vi "Length_5_R2.vi"() -> ()   [LabVIEW 2020]
uses:
  Support/Controls/Clst_Initialize Input.ctl
  Support/Controls/Clst_Result inspec.ctl
  Support/Controls/Cmd_Var Data IO.ctl
  Support/Controls/Cmd_Mouse Popup.ctl
  Variables/Global_Cal Info.vi
panel:
  in  "Measured 2":string[][](table) caption="잔류잡음측정"
  in  "Measured_ADJ":string[][](table) caption="조정후"
  out "최소범위":string
  in  "표시방식":string(combo)
  out "단위":string
  out "최대범위":string
  in  "Spec 변경":bool
  in  "Random":bool
  out "Resolution":string[][](table) caption="Spec"
  out "Spec":string[][](table)
  out "제목":string
  out "에러 출력":errorcluster
  out "Condition":string[][](table) caption="2. 직선성 시험"
  in  "최소눈금":string(combo)
  in  "Measured":string[][](table) caption="조정전"
  out "Load?":bool
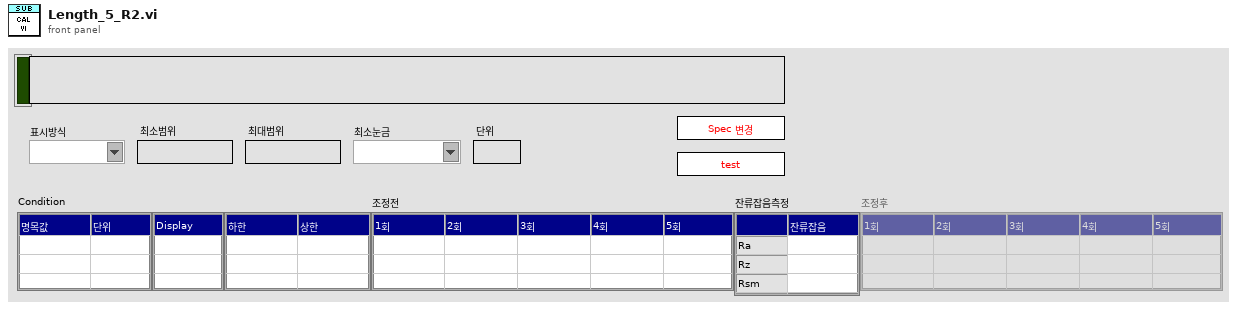
[diagram p1: front panel]
types:
  T1 = typedef "Cmd_Mouse Popup.ctl" = enum16{"활성화", "메뉴선택"}
  T2 = cluster{"Shift":bool, "Ctrl":bool, "Alt":bool, "Cmd":bool, "Opt":bool}
  T3 = typedef "Clst_Initialize Input.ctl" = cluster{"Initialize 1":cluster{"Condition":refnum<vi>[], "Spec":refnum<vi>[], "Measured":refnum<vi>[], "Resolution":refnum<vi>[], "Func_ext":string, "제목":refnum<vi>, "Measured_ADJ":refnum<vi>[]}, "Initialize 2":cluster{"문자열":refnum<vi>[], "콤보박스":refnum<vi>[], "링":refnum<vi>[], "열거형":refnum<vi>[], "테이블":refnum<vi>[], "여러열":refnum<vi>[], "디지털(DBL)":refnum<vi>[], "3D string":refnum<vi>[], "ctrl":refnum<vi>[], "boolean":refnum<vi>[]}}
  T4 = typedef "Clst_Result inspec.ctl" = cluster{"분해능":string, "문자열 1":string, "문자열 2":string, "숫자형 1":i32, "숫자형 2":i32, "숫자형 3":dbl, "문자배열 1D":string[], "문자배열 2D":string[][], "문자배열 3D":string[][][], "문자배열 4D":string[][][][], "불리언 1D":bool[]}
  T5 = typedef "Cmd_Var Data IO.ctl" = enum16{"Condition", "Condition Default", "Condition_Temp", "Resolution", "Resolution Default", "Resolution Old", "Spec", "Spec Default", "Spec Old", "Spec Temp", "Result", "Result2", "Result3", "Result_Temp", "Result_ADJ", "Result_ADJ2", "STD1", "STD2", "STD3", "STD4", "STD5", "STD Temp", "CMC", "CMC Default"}
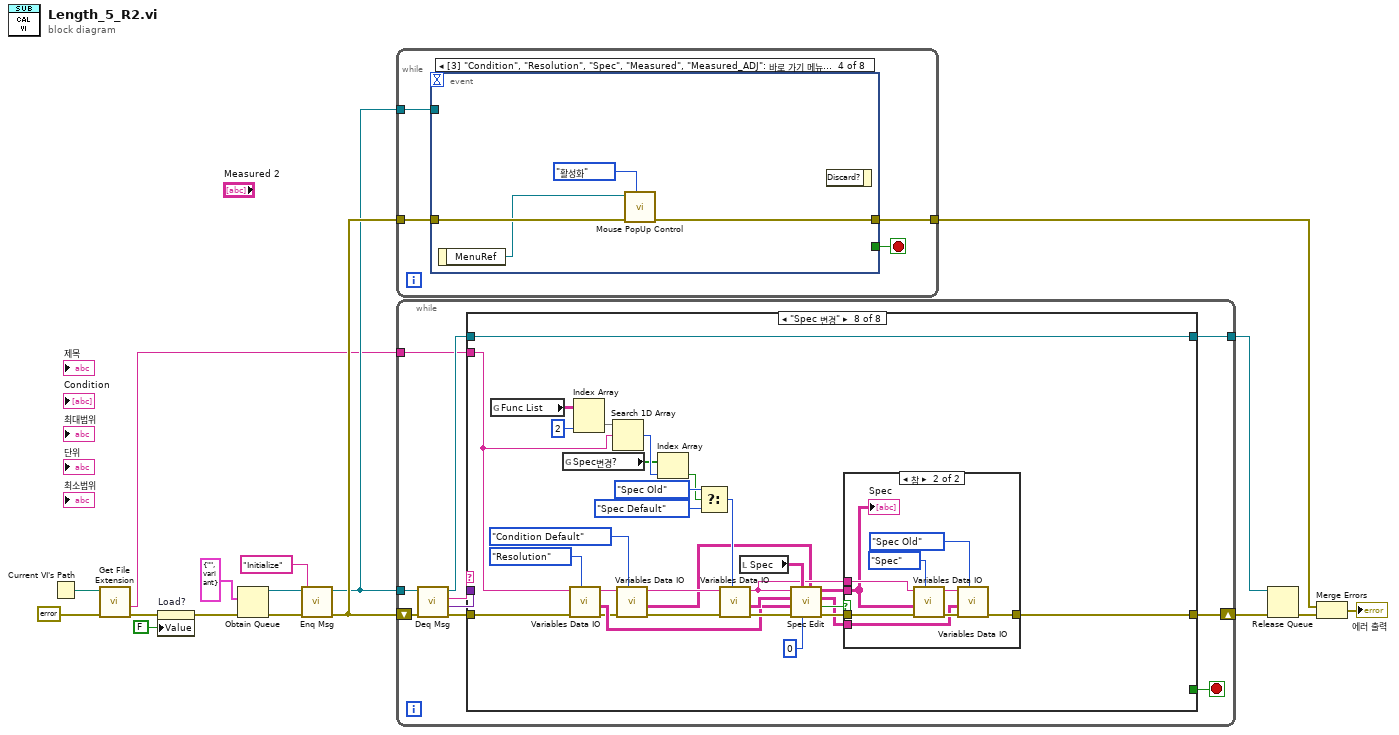
[diagram p0: block diagram]
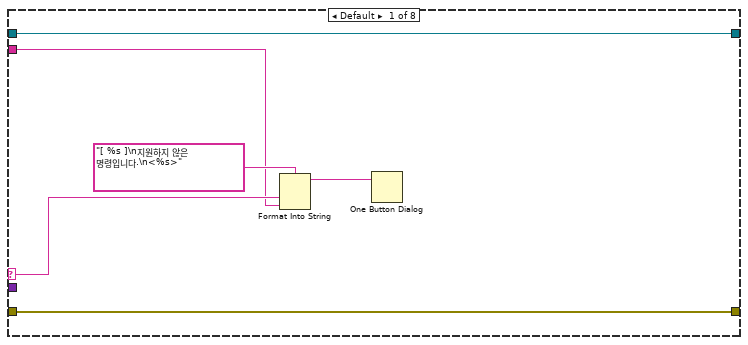
[diagram p2: hidden frame]
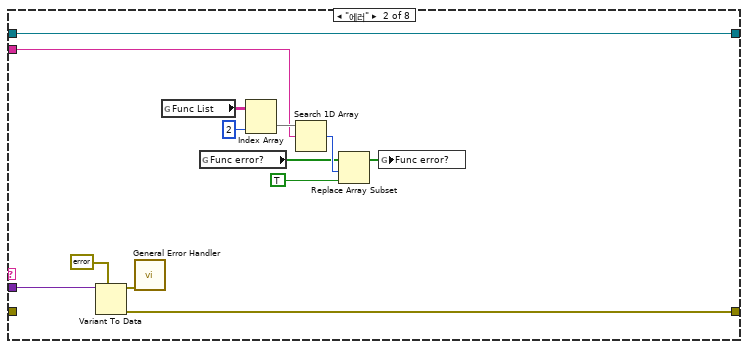
[diagram p3: hidden frame]
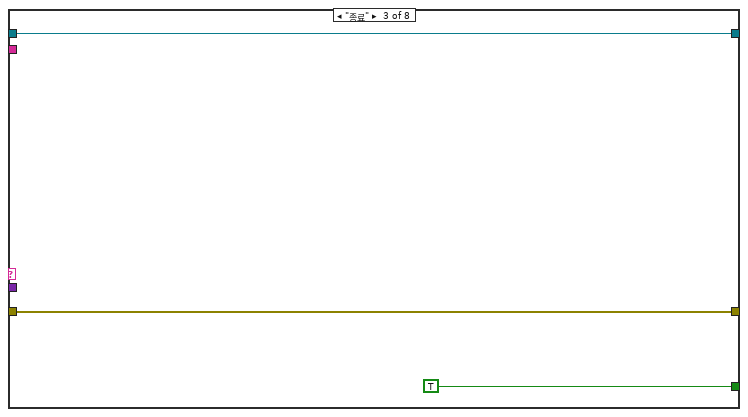
[diagram p4: hidden frame]
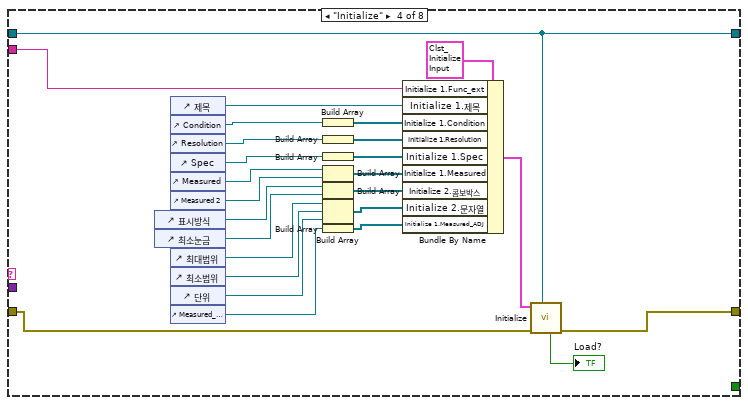
[diagram p5: hidden frame]
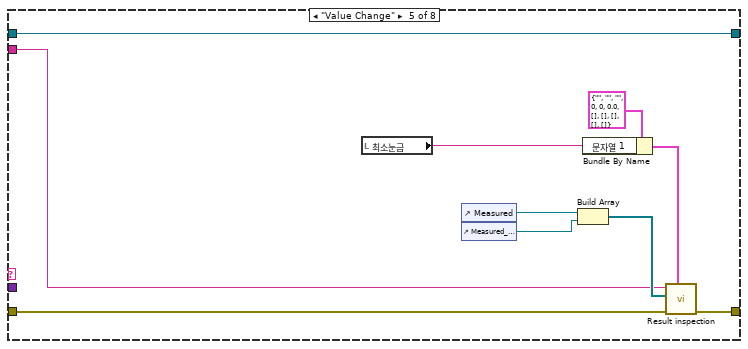
[diagram p6: hidden frame]
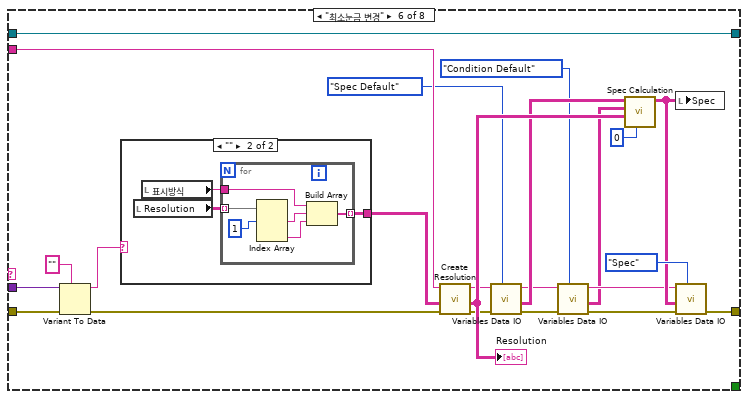
[diagram p7: hidden frame]
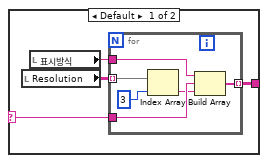
[diagram p8: hidden frame]
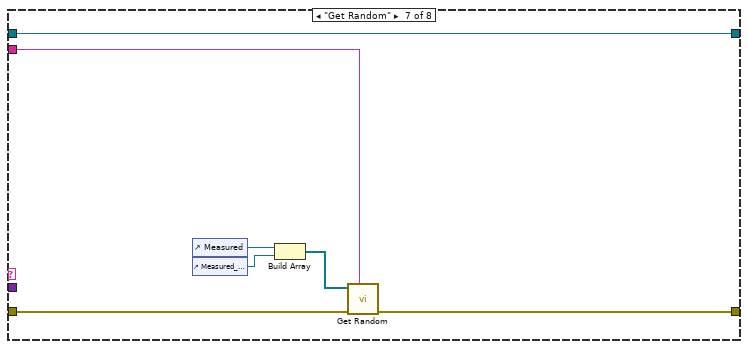
[diagram p9: hidden frame]
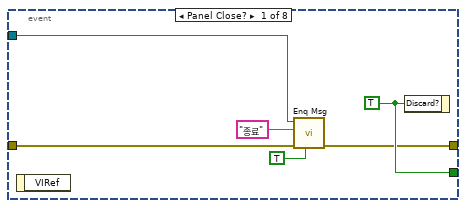
[diagram p11: hidden frame]
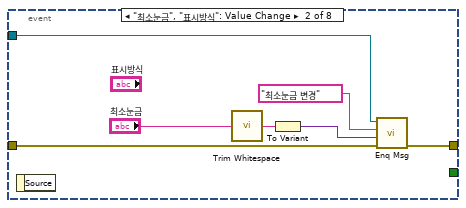
[diagram p12: hidden frame]
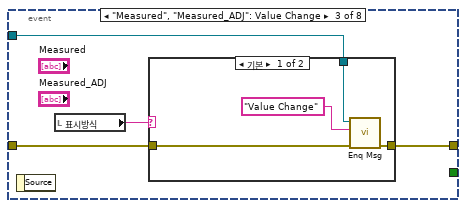
[diagram p13: hidden frame]
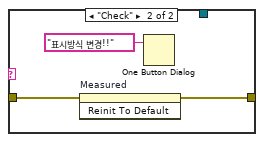
[diagram p14: hidden frame]
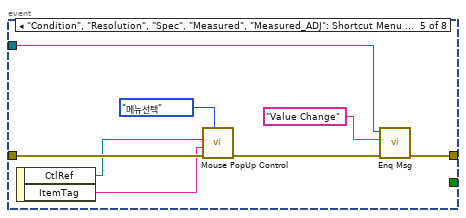
[diagram p15: hidden frame]
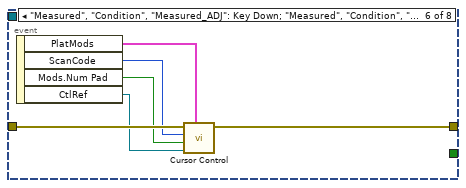
[diagram p16: hidden frame]
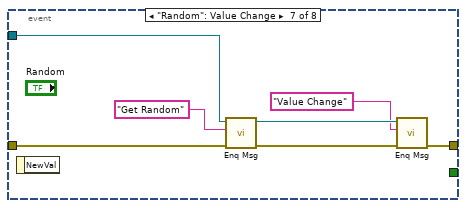
[diagram p17: hidden frame]
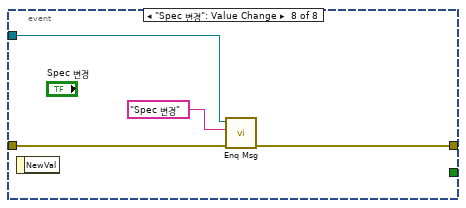
[diagram p18: hidden frame]
diagram:
  n1 = Current VI's Path() -> (path=w5:path)
  n2 = call <vilib>:"Get File Extension.vi"("error in (no error)"=errorcluster {"status"=FALSE, "code"=0, "source"=""} ("에러 상수"), "file"=w5) -> ("error out"=w3:errorcluster, "filename without extension"=w4:string)  [unwired: 5 in, 3 out]
  n3 = property on="Load?" class="Bool (엄격한)"(error in=w3, "Value"=FALSE ("Load?")) -> (error out=w2:errorcluster)  [unwired: 1 in, 1 out]
  n4 = Obtain Queue(element data type=cluster{"메세지":string, "값":variant} {"메세지"="", "값"=variant} ("Message Cluster"), error in (no error)=w2) -> (queue out=w14:refnum<queue>, error out=w16:errorcluster)  [unwired: 3 in, 1 out]
  n5 = call "Enq Msg.vi"("에러 입력(에러 없음)"=w16, "메세지"="Initialize", "큐 입력"=w14) -> ("에러 출력"=w15:errorcluster, "큐 출력"=w12:refnum<queue>)  [unwired: 7 in]
  n6 = while {
    tunnel: w15 -> [w19]
    tunnel: w12 -> [w20]
    tunnel: [w18] -> w9
    stop <- w21 stop-if-true
    n7 = event shown="[3] \"Condition\", \"Resolution\", \"Spec\", \"Measured\", \"Measured_ADJ\": 바로 가기 메뉴 활성화?" {
      selector: _ -> [_ _ _ _ _ _ _ _]
      dyn-events: _ -> [_ _ _ _ _ _ _ _]
      timeout: _ -> [_ _ _ _ _ _ _ _]
      tunnel: [w27 _ _ _ _ _ _ _] -> w21
      tunnel: w20 -> [w25 w33 w38 _ w50 _ w68 w72]
      tunnel: w19 -> [w26 w34 w36 w49 w57 w63 w69 w73]
      tunnel: [w23 w32 w37 w48 w51 w62 w64 w71] -> w18
      event Panel Close? {
        w27 = TRUE ("버림?")
        n8 = event-data() -> ()  [unwired: 1 in, 1 out]
        n9 = call "Enq Msg.vi"("우선순위 메시지?"=TRUE, "에러 입력(에러 없음)"=w26, "메세지"="종료", "큐 입력"=w25) -> ("에러 출력"=w23:errorcluster)  [unwired: 6 in, 1 out]
        n10 = event-data("Discard?"=w27) -> ()  [unwired: 1 in, 1 out]
      }
      event "최소눈금", "표시방식": Value Change {
        n11 = event-data() -> ()  [unwired: 1 in, 1 out]
        n12 = call <vilib>:"Trim Whitespace.vi"("string"="최소눈금") -> ("trimmed string"=w30:string)  [unwired: 1 in]
        n13 = To Variant(anything=w30) -> (Variant=w28:variant)
        n14 = call "Enq Msg.vi"("에러 입력(에러 없음)"=w34, "값"=w28, "메세지"="최소눈금 변경", "큐 입력"=w33) -> ("에러 출력"=w32:errorcluster)  [unwired: 6 in, 1 out]
      }
      event "Measured", "Measured_ADJ": Value Change {
        n15 = event-data() -> ()  [unwired: 1 in, 1 out]
        n16 = local read "표시방식"() -> (w35:string)
        n17 = case shown="기본" w35 {
          tunnel: w38 -> [w42 _]
          tunnel: [w41 w43] -> w37
          tunnel: w36 -> [w40 w44]
          frame Default {
            n18 = call "Enq Msg.vi"("에러 입력(에러 없음)"=w40, "메세지"="Value Change", "큐 입력"=w42) -> ("에러 출력"=w41:errorcluster)  [unwired: 7 in, 1 out]
          }
          frame "Check" {
            n19 = invoke on="Measured" class="Tbl (엄격한)" method="Reinit To Default"(error in=w44) -> (error out=w43:errorcluster)  [unwired: 2 in, 2 out]
            n20 = One Button Dialog(message="표시방식 변경!!" ("메시지")) -> ()  [unwired: 1 in, 1 out]
          }
        }
      }
      event "Condition", "Resolution", "Spec", "Measured", "Measured_ADJ": Shortcut Menu Activation? {
        n21 = event-data() -> ("MenuRef"=w47:refnum<k9>)  [unwired: 1 in]
        n22 = call "Mouse PopUp Control.vi"("type"=Cmd_Mouse_Popup."활성화", "error in"=w49, "메뉴 참조"=w47) -> ("error out"=w48:errorcluster)  [unwired: 8 in]
        n23 = event-data() -> ()  [unwired: 2 in, 1 out]
      }
      event "Condition", "Resolution", "Spec", "Measured", "Measured_ADJ": Shortcut Menu Selection (User) {
        n24 = event-data() -> ("CtlRef"=w55:refnum<vi>, "ItemTag"=w54:string)  [unwired: 1 in]
        n25 = call "Mouse PopUp Control.vi"("type"=Cmd_Mouse_Popup."메뉴선택", "error in"=w57, "아이템 태그"=w54, "Tbl 참조 번호"=w55) -> ("error out"=w52:errorcluster)  [unwired: 7 in]
        n26 = call "Enq Msg.vi"("에러 입력(에러 없음)"=w52, "메세지"="Value Change", "큐 입력"=w50) -> ("에러 출력"=w51:errorcluster)  [unwired: 7 in, 1 out]
      }
      event "Measured", "Condition", "Measured_ADJ": Key Down; "Measured", "Condition", "Measured_ADJ": Key Repeat {
        n27 = event-data() -> ("PlatMods"=w58:T2, "ScanCode"=w61:i16, "Mods.Num Pad"=w60:bool, "CtlRef"=w59:refnum<vi>)  [unwired: 1 in]
        n28 = call "Cursor Control.vi"("플랫폼 조합키"=w58, "참조"=w59, "Num Pad"=w60, "ScanCode"=w61, "error in"=w63) -> ("error out"=w62:errorcluster)  [unwired: 5 in, 1 out]
      }
      event "Random": Value Change {
        n29 = event-data() -> ()  [unwired: 1 in, 1 out]
        n30 = call "Enq Msg.vi"("에러 입력(에러 없음)"=w69, "메세지"="Get Random", "큐 입력"=w68) -> ("에러 출력"=w67:errorcluster, "큐 출력"=w66:refnum<queue>)  [unwired: 7 in]
        n31 = call "Enq Msg.vi"("에러 입력(에러 없음)"=w67, "메세지"="Value Change", "큐 입력"=w66) -> ("에러 출력"=w64:errorcluster)  [unwired: 7 in, 1 out]
      }
      event "Spec 변경": Value Change {
        n32 = event-data() -> ()  [unwired: 1 in, 1 out]
        n33 = call "Enq Msg.vi"("에러 입력(에러 없음)"=w73, "메세지"="Spec 변경", "큐 입력"=w72) -> ("에러 출력"=w71:errorcluster)  [unwired: 7 in, 1 out]
      }
    }
  }
  n34 = while {
    shift-right: [w84] -> w11
    shift-left: w15 -> [w83]
    tunnel: w12 -> [w81]
    tunnel: [w76] -> w10
    tunnel: w4 -> [w75]
    stop <- w77 stop-if-true
    n35 = call "Deq Msg.vi"("에러 입력(에러 없음)"=w83, "큐 입력"=w81) -> ("에러 출력"=w82:errorcluster, "값"=w78:variant, "메세지"=w80:string, "큐 출력"=w79:refnum<queue>)  [unwired: 6 in]
    n36 = case shown="\"Spec 변경\"" w80 {
      selector: w80 -> [w86 _ _ _ _ _ _ _]
      tunnel: w82 -> [w90 _ w106 w132 w136 w164 w187 w214]
      tunnel: [w90 w100 w106 w122 w141 w157 w188 w217] -> w84
      tunnel: w79 -> [w89 w99 w104 w116 w142 w165 w191 w221]
      tunnel: w78 -> [_ w101 _ _ _ w163 _ _]
      tunnel: [_ _ TRUE ("버림?") _ _ _ _ _] -> w77
      tunnel: [w89 w99 w104 w116 w142 w165 w191 w221] -> w76
      tunnel: w75 -> [w85 w91 _ w117 w135 w161 w186 w199]
      frame Default {
        n37 = Format Into String(format string="[ %s ]\n지원하지 않은 명령입니다.\n<%s>" ("메시지"), w86, w85) -> (resulting string=w87:string)  [unwired: 2 in, 1 out]
        n38 = One Button Dialog(message=w87) -> ()  [unwired: 1 in, 1 out]
      }
      frame "에러" {
        n39 = Variant To Data(type=errorcluster {"status"=FALSE, "code"=0, "source"=""} ("에러 출력"), Variant=w101) -> (data=w103:errorcluster, error out=w100:errorcluster)  [unwired: 1 in]
        n40 = call <vilib>:"General Error Handler.vi"("error in (no error)"=w103) -> ()  [unwired: 10 in, 5 out]
        n41 = global read "Global_Cal Info.vi" "Func List"() -> (w93:string[][])
        n42 = global read "Global_Cal Info.vi" "Func error?"() -> (w96:bool[])
        n43 = Index Array(array=w93, index (col)=2 ("비활성화된 인덱스 (열)")) -> (element=w94:string[])  [unwired: 1 in]
        n44 = Search 1D Array(1D array=w94, element=w91) -> (index of element=w97:i32)  [unwired: 1 in]
        n45 = Replace Array Subset(array=w96, new element=TRUE ("새 원소/부분배열"), index=w97) -> (w98:bool[])
        n46 = global write "Global_Cal Info.vi" "Func error?"(w98) -> ()
      }
      frame "종료" {
      }
      frame "Initialize" {
        n47 = control-ref of="표시방식"() -> (w115:refnum<vi>)
        n48 = control-ref of="최소눈금"() -> (w125:refnum<vi>)
        n49 = control-ref of="제목"() -> (w123:refnum<vi>)
        n50 = control-ref of="Condition"() -> (w129:refnum<vi>)
        n51 = control-ref of="Resolution"() -> (w118:refnum<vi>)
        n52 = control-ref of="Spec"() -> (w121:refnum<vi>)
        n53 = control-ref of="Measured"() -> (w126:refnum<vi>)
        n54 = control-ref of="Measured 2"() -> (w107:refnum<vi>)
        n55 = control-ref of="최대범위"() -> (w111:refnum<vi>)
        n56 = control-ref of="최소범위"() -> (w112:refnum<vi>)
        n57 = control-ref of="단위"() -> (w114:refnum<vi>)
        n58 = control-ref of="Measured_ADJ"() -> (w109:refnum<vi>)
        n59 = Build Array(w129) -> (w128:refnum<vi>[])
        n60 = Build Array(w118) -> (w119:refnum<vi>[])
        n61 = Build Array(w121) -> (w120:refnum<vi>[])
        n62 = Build Array(w126, w107) -> (w127:refnum<vi>[])
        n63 = Build Array(w115, w125) -> (w124:refnum<vi>[])
        n64 = Build Array(w111, w112, w114) -> (w113:refnum<vi>[])
        n65 = Build Array(w109) -> (w108:refnum<vi>[])
        n66 = Bundle By Name(cluster=T3 {"Initialize 1"={"Condition"=[], "Spec"=[], "Measured"=[], "Resolution"=[], "Func_ext"="", "제목"=refnum, "Measured_ADJ"=[]}, "Initialize 2"={"문자열"=[], "콤보박스"=[], "링"=[], "열거형"=[], "테이블"=[], "여러열"=[], "디지털(DBL)"=[], "3D string"=[], "ctrl"=[], "boolean"=[]}} ("입력 클러스터"), "Initialize 1.Func_ext"=w117, "Initialize 1.제목"=w123, "Initialize 1.Condition"=w128, "Initialize 1.Resolution"=w119, "Initialize 1.Spec"=w120, "Initialize 1.Measured"=w127, "Initialize 2.콤보박스"=w124, "Initialize 2.문자열"=w113, "Initialize 1.Measured_ADJ"=w108) -> (w130:T3)
        n67 = call "Initialize.vi"("큐 입력"=w116, "error in"=w132, "입력 클러스터"=w130) -> ("error out"=w122:errorcluster, "Load?"=→"Load?":bool)  [unwired: 5 in, 2 out]
      }
      frame "Value Change" {
        n68 = local read "최소눈금"() -> (w134:string)
        n69 = control-ref of="Measured"() -> (w140:refnum<vi>)
        n70 = control-ref of="Measured_ADJ"() -> (w133:refnum<vi>)
        n71 = Build Array(w140, w133) -> (w139:refnum<vi>[])
        n72 = Bundle By Name(cluster=T4 {"분해능"="", "문자열 1"="", "문자열 2"="", "숫자형 1"=0, "숫자형 2"=0, "숫자형 3"=0.0, "문자배열 1D"=[], "문자배열 2D"=[], "문자배열 3D"=[], "문자배열 4D"=[], "불리언 1D"=[]} ("입력 클러스터"), "문자열 1"=w134) -> (w137:T4)
        n73 = call "Result inspection.vi"("입력 클러스터"=w137, "error in"=w136, "Ref. Data (Inspection)"=w139, "Func ext"=w135) -> ("error out"=w141:errorcluster)  [unwired: 4 in, 3 out]
      }
      frame "최소눈금 변경" {
        n74 = Variant To Data(error in=w164, type="", Variant=w163) -> (data=w150:string, error out=w152:errorcluster)
        n75 = case shown="\"\"" w150 {
          selector: w150 -> [w166 _]
          tunnel: [w169 w178] -> w151
          frame Default {
            n76 = local read "Resolution"() -> (w168:string[][])
            n77 = local read "표시방식"() -> (w167:string)
            n78 = for {
              tunnel: w168 -> [w175] mode=indexing
              tunnel: w166 -> [w174]
              tunnel: [w172] -> w169 mode=indexing
              tunnel: w167 -> [w171]
              n79 = Index Array(array=w175, index=3 ("인덱스")) -> (element=w173:string)
              n80 = Build Array(w171, w174, w173) -> (w172:string[])
            }
          }
          frame "" {
            n81 = local read "Resolution"() -> (w177:string[][])
            n82 = local read "표시방식"() -> (w176:string)
            n83 = for {
              tunnel: w177 -> [w184] mode=indexing
              tunnel: [w183] -> w178 mode=indexing
              tunnel: w176 -> [w182]
              n84 = Index Array(array=w184, index #1=1 ("인덱스")) -> (element #1=w180:string, element #3=w179:string)  [unwired: 2 in, 1 out]
              n85 = Build Array(w182, w180, w179) -> (w183:string[])
            }
          }
        }
        n86 = call "Create Resolution.vi"("에러 입력(에러 없음)"=w152, "Resolution"=w151, "Func_ext"=w161) -> ("에러 출력"=w155:errorcluster, "Resolution Out"=w158:string[][], "Func_ext 출력"=w154:string)  [unwired: 6 in]
        "Resolution" <- w158
        n87 = call "Variables Data IO.vi"("Select"=Cmd_Var_Data_IO."Spec Default", "error in"=w155, "Func_ext"=w154) -> ("error out"=w146:errorcluster, "Data Out"=w153:string[][], "Func_ext Out"=w147:string)  [unwired: 6 in]
        n88 = call "Variables Data IO.vi"("Select"=Cmd_Var_Data_IO."Condition Default", "error in"=w146, "Func_ext"=w147) -> ("error out"=w144:errorcluster, "Data Out"=w143:string[][], "Func_ext Out"=w145:string)  [unwired: 6 in]
        n89 = call "Spec Calculation.vi"("기준값 열번호"=0 ("열번호(기준값)"), "Resolution"=w158, "Condition in"=w143, "Spec Default"=w153) -> ("Spec out"=w149:string[][])  [unwired: 6 in, 1 out]
        n90 = local write "Spec"(w149) -> ()
        n91 = call "Variables Data IO.vi"("Select"=Cmd_Var_Data_IO."Spec", "error in"=w144, "Data In"=w149, "Func_ext"=w145) -> ("error out"=w157:errorcluster)  [unwired: 5 in, 2 out]
      }
      frame "Get Random" {
        n92 = control-ref of="Measured"() -> (w190:refnum<vi>)
        n93 = control-ref of="Measured_ADJ"() -> (w185:refnum<vi>)
        n94 = Build Array(w190, w185) -> (w189:refnum<vi>[])
        n95 = call "Get Random.vi"("Func_Ext"=w186, "에러 입력"=w187, "Meas"=w189) -> ("에러 출력"=w188:errorcluster)  [unwired: 7 in, 1 out]
      }
      frame "Spec 변경" {
        n96 = global read "Global_Cal Info.vi" "Func List"() -> (w204:string[][])
        n97 = global read "Global_Cal Info.vi" "Spec변경?"() -> (w200:bool[])
        n98 = call "Variables Data IO.vi"("Select"=Cmd_Var_Data_IO."Resolution", "error in"=w214, "Func_ext"=w199) -> ("error out"=w197:errorcluster, "Data Out"=w208:string[][], "Func_ext Out"=w195:string)  [unwired: 6 in]
        n99 = Index Array(array=w204, index (col)=2 ("비활성화된 인덱스 (열)")) -> (element=w202:string[])  [unwired: 1 in]
        n100 = Search 1D Array(1D array=w202, element=w199) -> (index of element=w201:i32)  [unwired: 1 in]
        n101 = call "Variables Data IO.vi"("Select"=Cmd_Var_Data_IO."Condition Default", "error in"=w197, "Func_ext"=w195) -> ("error out"=w196:errorcluster, "Data Out"=w192:string[][], "Func_ext Out"=w194:string)  [unwired: 6 in]
        n102 = Index Array(array=w200, index=w201) -> (element=w205:bool)
        n103 = Select(t=Cmd_Var_Data_IO."Spec Old" ("Select"), s=w205, f=Cmd_Var_Data_IO."Spec Default" ("Select")) -> (s? t:f=w198:T5)
        n104 = call "Variables Data IO.vi"("Select"=w198, "error in"=w196, "Func_ext"=w194) -> ("error out"=w216:errorcluster, "Data Out"=w209:string[][], "Func_ext Out"=w210:string)  [unwired: 6 in]
        n105 = local read "Spec"() -> (w211:string[][])
        n106 = call "Spec Edit.vi"("Condition"=w192, "열번호(기준값)"=0, "Spec Value"=w211, "에러 입력(에러 없음)"=w216, "Resolution"=w208, "Spec Default"=w209, "Func_ext"=w210) -> ("에러 출력"=w218:errorcluster, "변경?"=w219:bool, "Spec Default out"=w213:string[][], "Spec 출력"=w220:string[][])  [unwired: 1 in]
        n107 = case shown="참" w219 {
          tunnel: w220 -> [_ w228]
          tunnel: w218 -> [w222 w231]
          tunnel: [w222 w226] -> w217
          tunnel: w210 -> [_ w229]
          tunnel: w213 -> [_ w224]
          frame False {
          }
          frame True {
            n108 = call "Variables Data IO.vi"("Select"=Cmd_Var_Data_IO."Spec", "error in"=w231, "Data In"=w228, "Func_ext"=w229) -> ("error out"=w227:errorcluster, "Func_ext Out"=w225:string)  [unwired: 5 in, 1 out]
            n109 = call "Variables Data IO.vi"("Select"=Cmd_Var_Data_IO."Spec Old", "error in"=w227, "Data In"=w224, "Func_ext"=w225) -> ("error out"=w226:errorcluster)  [unwired: 5 in, 2 out]
            "Spec" <- w228
          }
        }
      }
    }
  }
  n110 = Release Queue(queue=w10, error in (no error)=w11) -> (error out=w8:errorcluster)  [unwired: 1 in, 2 out]
  n111 = Merge Errors(w9, w8) -> (→"에러 출력":errorcluster)
